vi "Save Image.vi"(8 "error in (no error)":errorcluster, 11 "Save Image in":refnum<class "Save Image.lvclass">) -> (0 "error out":errorcluster, 3 "Save Image out":refnum<class "Save Image.lvclass">)   [LabVIEW 2018, in "Save Image.lvclass"]
uses:
  Save Image.lvclass
  Save Image.lvclass/Save Image.ctl
  <userlib>/gfitsio/gfitsio-write-image-subset-variant.vi
  <userlib>/gfitsio/gfitsio.lvlib
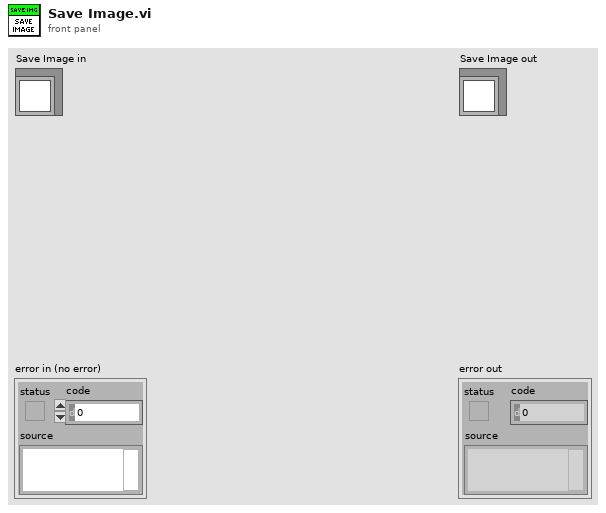
[diagram p1: front panel]
types:
  T1 = typedef "gfitsio.lvlib/gfitsio-refnum.ctl" = refnum<k1>
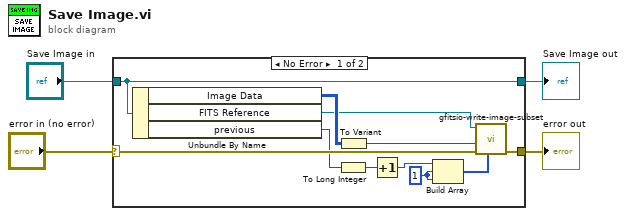
[diagram p0: block diagram]
diagram:
  n1 = case shown="No Error" "error in (no error)" {
    selector: "error in (no error)" -> [w15 w17]
    tunnel: [w12 w17] -> w2
    tunnel: "Save Image in" -> [w11 w16]
    tunnel: [w11 w16] -> w1
    frame No Error {
      w10 = 1
      n2 = Unbundle By Name(w11) -> ("Image Data"=w14:u16[][][], "FITS Reference"=w8:T1, "previous"=w6:u16)
      n3 = To Long Integer(number=w6) -> (32bit integer=w5:i32)
      n4 = To Variant(anything=w14) -> (Variant=w13:variant)
      n5 = Increment(x=w5) -> (x+1=w7:i32)
      n6 = Build Array(w7, w10, w10) -> (w9:i32[])
      n7 = call-poly <userlib>:"gfitsio-write-image-subset.vi"("fpixel"=w9, "error in (no error)"=w15, "data"=w13, "gfits refnum"=w8) -> ("error out"=w12:errorcluster)  [unwired: 6 in, 1 out]
    }
    frame Error {
    }
  }
  "error out" <- w2
  "Save Image out" <- w1
